vi "auto vison.vi"(3 "error in (no error)":errorcluster, 4 "Image Src":T1) -> (0 "error out":errorcluster, 1 "TOO FAR":bool, 2 "There":bool)   [LabVIEW 2014]
uses:
  <vilib>/vision/Image Controls.llb/IMAQ Image.ctl
  <vilib>/vision/NI_Vision_Development_Module.lvlib
panel:
  out "y1":dbl
  out "Image Out 2":T1(plugin-control)
  out "error out 2":errorcluster
  out "Image":T1(plugin-control)
  in  "Blue or Luma or Val or Inten Range (Find Ls)":cluster{"Lower value":i32, "Upper value":i32}={"Lower value"=84, "Upper value"=255}
  in  "Green or Sat Range (Find Ls)":cluster{"Lower value":i32, "Upper value":i32}={"Lower value"=193, "Upper value"=255}
  in  "Red or Hue Range (Find Ls)":cluster{"Lower value":i32, "Upper value":i32}={"Lower value"=79, "Upper value"=255}
  out "Image Out":T1
  out "Number of Edges (L right)":i32
  out "Edges Coordinates (L right)":cluster{"X":sgl, "Y":sgl}[](array[cluster]) {"Y" format="%.2f"; "X" format="%.2f"}
  out "Number of Edges (L left)":i32
  out "Edges Coordinates (L left)":cluster{"X":sgl, "Y":sgl}[](array[cluster]) {"Y" format="%.2f"; "X" format="%.2f"}
  out "Number of Edges (Ltop)":i32
  out "Edges Coordinates (Ltop)":cluster{"X":sgl, "Y":sgl}[](array[cluster]) {"Y" format="%.2f"; "X" format="%.2f"}
types:
  T1 = typedef "IMAQ Image.ctl" = refnum<image>
  T2 = enum16{"Get First Edge", "Get First + Last Edge", "Get All Edges"}
  T3 = cluster{"Level Type":enum32{"Absolute Value", "Relative value"}, "Threshold Level":i32, "Hysteresis":i32}
  T4 = enum32{"AutoM", "Close", "Dilate", "Erode", "Gradient", "Gradient out", "Gradient in", "Hit miss", "Open", "PClose", "POpen", "Thick", "Thin"}
  T5 = cluster{"Brightness":sgl, "Contrast":sgl, "Gamma":sgl}
  T6 = cluster{"Global Rectangle":i32[], "Contours":cluster{"ID":enum32{"External", "Internal"}, "Type":u32, "Coordinates":i32[]}[]}
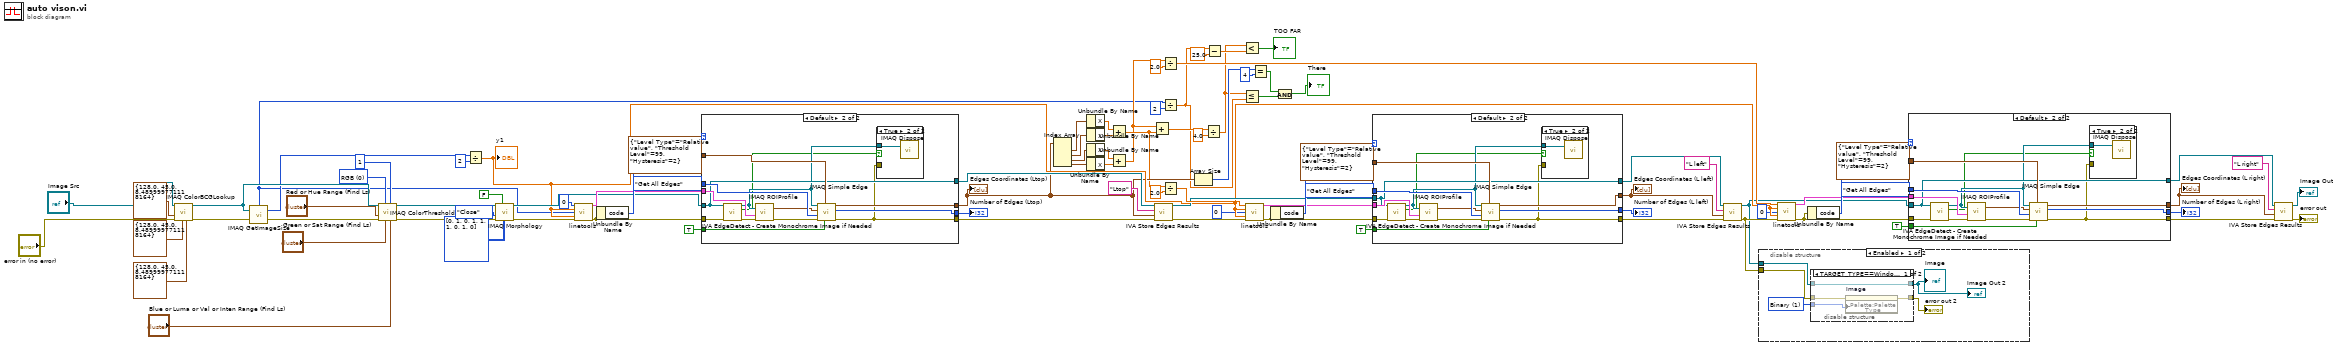
[diagram p0: block diagram]
diagram:
  w89 = u16 0 items=["RGB", "HSL", "HSV", "HSI"] ("Color Mode")
  n1 = call "IMAQ ColorBCGLookup"("Blue BCG Values"=T5 {"Brightness"=128.0, "Contrast"=45.0, "Gamma"=8.49}, "Green BCG Values"=T5 {"Brightness"=128.0, "Contrast"=45.0, "Gamma"=8.49}, "error in (no error)"="error in (no error)", "Red BCG Values"=T5 {"Brightness"=128.0, "Contrast"=45.0, "Gamma"=8.49}, "Image Src"="Image Src") -> ("error out"=w36:errorcluster, "Image Dst Out"=w56:T1)  [unwired: 2 in, 3 out]
  n2 = call "IMAQ GetImageSize"("Image"=w56, "error in (no error)"=w36) -> ("Y Resolution"=w49:i32, "X Resolution"=w14:i32, "error out"=w55:errorcluster)  [unwired: 2 in]
  n3 = call "IMAQ ColorThreshold"("Blue or Luma or Val or Inten Range"="Blue or Luma or Val or Inten Range (Find Ls)", "Replace Value"=1, "Green or Sat Range"="Green or Sat Range (Find Ls)", "Color Mode"=w89, "error in (no error)"=w55, "Red or Hue Range"="Red or Hue Range (Find Ls)", "Image Src"=w56) -> ("error out"=w34:errorcluster, "Image Dst Out"=w35:T1)  [unwired: 1 in, 2 out]
  n4 = Divide(x=w49, y=2) -> (x/y=w26:dbl)
  "y1" <- w26
  n5 = call "IMAQ Morphology"("Structuring Element"=i32[][] [[0, 1, 0], [1, 1, 1], [0, 1, 0]], "Square/Hexa (Square)"=FALSE, "error in (no error)"=w34, "Operation"=T4."Close", "Image Src"=w35) -> ("error out"=w47:errorcluster, "Image Dst Out"=w28:T1)  [unwired: 2 in, 3 out]
  n6 = call "linetools.vi"("X1"=0, "Y1"=w26, "X2"=w14, "Y2"=w26, "error in (no error)"=w47) -> ("output cluster"=w48:T6, "error out"=w29:errorcluster)  [unwired: 9 in]
  n7 = Unbundle By Name(w29) -> ("code"=w77:i32)
  n8 = case shown="Default" w77 {
    tunnel: T3 {"Level Type"=enum."Relative value", "Threshold Level"=99, "Hysteresis"=2} ("Threshold Parameters") -> [_ w108]
    tunnel: T2."Get All Edges" ("Process") -> [_ w107]
    tunnel: [_ w106] -> w80
    tunnel: w29 -> [_ w99]
    tunnel: w28 -> [w94 w100]
    tunnel: [_ w103] -> w20
    tunnel: [_ w95] -> w78
    tunnel: w48 -> [_ w102]
    tunnel: TRUE ("Sub-Pixel Accuracy") -> [_ w101]
    tunnel: [w94 w100] -> w75
    frame -1074396199, -1074396198 {
      # "Discard Coordinate System Error"
    }
    frame Default {
      n9 = call <vilib>:"IVA EdgeDetect - Create Monochrome Image if Needed.vi"("error in (no error)"=w99, "Image In"=w100) -> ("error out"=w98:errorcluster, "Mono Image Created"=w96:bool, "Mono Image Out"=w97:T1)  [unwired: 7 out]
      n10 = call "IMAQ ROIProfile"("error in (no error)"=w98, "ROI Descriptor"=w102, "Image"=w97) -> ("error out"=w104:errorcluster, "Pixel Coordinates"=w105:cluster{"X":u32, "Y":u32}[])  [unwired: 4 out]
      n11 = call "IMAQ Simple Edge"("Sub-Pixel Accuracy"=w101, "Threshold Parameters"=w108, "error in (no error)"=w104, "Process"=w107, "Pixel Coordinates"=w105, "Image Src"=w97) -> ("error out"=w95:errorcluster, "Number of Edges"=w106:i32, "Edges Coordinates"=w103:cluster{"X":sgl, "Y":sgl}[])  [unwired: 3 out]
      n12 = case shown="True" w96 {
        tunnel: w97 -> [_ w109]
        tunnel: w95 -> [_ _]
        frame False {
        }
        frame True {
          n13 = call "IMAQ Dispose"("Image"=w109) -> ()  [unwired: 2 in, 4 out]
        }
      }
    }
  }
  "Edges Coordinates (Ltop)" <- w20
  "Number of Edges (Ltop)" <- w80
  n14 = Index Array(array=w20) -> (element #1=w53:cluster{"X":sgl, "Y":sgl}, element #2=w52:cluster{"X":sgl, "Y":sgl}, element #3=w54:cluster{"X":sgl, "Y":sgl}, element #4=w51:cluster{"X":sgl, "Y":sgl})  [unwired: 4 in]
  n15 = Unbundle By Name(w53) -> ("X"=w19:sgl)
  n16 = Unbundle By Name(w52) -> ("X"=w46:sgl)
  n17 = Unbundle By Name(w54) -> ("X"=w45:sgl)
  n18 = Unbundle By Name(w51) -> ("X"=w44:sgl)
  n19 = Add(x=w19, y=w46) -> (x+y=w18:sgl)
  n20 = Add(x=w45, y=w44) -> (x+y=w17:sgl)
  n21 = Add(x=w17, y=w18) -> (x+y=w16:sgl)
  n22 = call <vilib>:"IVA Store Edges Results.vi"("error in (no error)"=w78, "Edge Coordinates"=w20, "Step Name"="Ltop", "Image in"=w75) -> ("error out"=w42:errorcluster, "Image dup"=w32:T1)  [unwired: 6 out]
  n23 = Divide(x=w17, y=sgl 2.0) -> (x/y=w27:sgl)
  n24 = Divide(x=w14, y=2) -> (x/y=w6:dbl)
  n25 = Divide(x=w18, y=sgl 2.0) -> (x/y=w41:sgl)
  n26 = Array Size(array=w20) -> (size(s)=w11:i32)
  n27 = Divide(x=w16, y=sgl 4.0) -> (x/y=w4:sgl)
  n28 = Subtract(x=w6, y=25.0) -> (x-y=w5:dbl)
  n29 = Less?(x=w4, y=w5) -> (x < y?=→"TOO FAR":bool)
  n30 = Less Or Equal?(x=w4, y=w6) -> (x <= y?=w12:bool)
  n31 = call "linetools.vi"("X1"=w41, "Y1"=w26, "X2"=0, "Y2"=w26, "error in (no error)"=w42) -> ("output cluster"=w43:T6, "error out"=w31:errorcluster)  [unwired: 9 in]
  n32 = Equal?(x=w11, y=4) -> (x = y?=w9:bool)
  n33 = Unbundle By Name(w31) -> ("code"=w68:i32)
  n34 = And(x=w9, y=w12) -> (x .and. y?=→"There":bool)
  n35 = case shown="Default" w68 {
    tunnel: T3 {"Level Type"=enum."Relative value", "Threshold Level"=99, "Hysteresis"=2} ("Threshold Parameters") -> [_ w124]
    tunnel: T2."Get All Edges" ("Process") -> [_ w123]
    tunnel: [_ w122] -> w72
    tunnel: w31 -> [_ w115]
    tunnel: w32 -> [w110 w116]
    tunnel: [_ w119] -> w70
    tunnel: [_ w111] -> w69
    tunnel: w43 -> [_ w118]
    tunnel: TRUE ("Sub-Pixel Accuracy") -> [_ w117]
    tunnel: [w110 w116] -> w66
    frame -1074396199, -1074396198 {
      # "Discard Coordinate System Error"
    }
    frame Default {
      n36 = call <vilib>:"IVA EdgeDetect - Create Monochrome Image if Needed.vi"("error in (no error)"=w115, "Image In"=w116) -> ("error out"=w114:errorcluster, "Mono Image Created"=w112:bool, "Mono Image Out"=w113:T1)  [unwired: 7 out]
      n37 = call "IMAQ ROIProfile"("error in (no error)"=w114, "ROI Descriptor"=w118, "Image"=w113) -> ("error out"=w120:errorcluster, "Pixel Coordinates"=w121:cluster{"X":u32, "Y":u32}[])  [unwired: 4 out]
      n38 = call "IMAQ Simple Edge"("Sub-Pixel Accuracy"=w117, "Threshold Parameters"=w124, "error in (no error)"=w120, "Process"=w123, "Pixel Coordinates"=w121, "Image Src"=w113) -> ("error out"=w111:errorcluster, "Number of Edges"=w122:i32, "Edges Coordinates"=w119:cluster{"X":sgl, "Y":sgl}[])  [unwired: 3 out]
      n39 = case shown="True" w112 {
        tunnel: w113 -> [_ w125]
        tunnel: w111 -> [_ _]
        frame False {
        }
        frame True {
          n40 = call "IMAQ Dispose"("Image"=w125) -> ()  [unwired: 2 in, 4 out]
        }
      }
    }
  }
  "Edges Coordinates (L left)" <- w70
  "Number of Edges (L left)" <- w72
  n41 = call <vilib>:"IVA Store Edges Results.vi"("error in (no error)"=w69, "Edge Coordinates"=w70, "Step Name"="L left", "Image in"=w66) -> ("error out"=w33:errorcluster, "Image dup"=w24:T1)  [unwired: 6 out]
  n42 = disable-structure shown="Enabled" {
    disable-tunnel: w33 -> [w127 _]
    disable-tunnel: w24 -> [w126 _]
    frame Enabled {
      w129 = u32 1 items=["Grayscale", "Binary", "Gradient", "Rainbow", "Temperature", "User Defined"] ("Palette")
      n43 = disable-structure "Conditional Disable Structure" shown="TARGET_TYPE==Windows" {
        disable-tunnel: w127 -> [w134 w135]
        disable-tunnel: [w133 w135] -> w130
        disable-tunnel: w126 -> [w132 w136]
        disable-tunnel: [w132 w136] -> w128
        disable-tunnel: w129 -> [w131 _]
        frame condition #0 {
          n44 = property on="Image" class="ImageControl"(error in=w134, "Palette:Palette Type"=w131) -> (error out=w133:errorcluster)  [unwired: 1 in, 1 out]
        }
        frame condition #1 (active) {
        }
      }
      "Image" <- w128
      "error out 2" <- w130
      "Image Out 2" <- w128
    }
    frame Disabled {
    }
  }
  n45 = call "linetools.vi"("X1"=w27, "Y1"=w26, "X2"=0, "Y2"=w26, "error in (no error)"=w33) -> ("output cluster"=w38:T6, "error out"=w23:errorcluster)  [unwired: 9 in]
  n46 = Unbundle By Name(w23) -> ("code"=w59:i32)
  n47 = case shown="Default" w59 {
    tunnel: T3 {"Level Type"=enum."Relative value", "Threshold Level"=99, "Hysteresis"=2} ("Threshold Parameters") -> [_ w151]
    tunnel: T2."Get All Edges" ("Process") -> [_ w150]
    tunnel: [_ w149] -> w63
    tunnel: w23 -> [_ w142]
    tunnel: w24 -> [w137 w143]
    tunnel: [_ w146] -> w21
    tunnel: [_ w138] -> w61
    tunnel: w38 -> [_ w145]
    tunnel: TRUE ("Sub-Pixel Accuracy") -> [_ w144]
    tunnel: [w137 w143] -> w57
    frame -1074396199, -1074396198 {
      # "Discard Coordinate System Error"
    }
    frame Default {
      n48 = call <vilib>:"IVA EdgeDetect - Create Monochrome Image if Needed.vi"("error in (no error)"=w142, "Image In"=w143) -> ("error out"=w141:errorcluster, "Mono Image Created"=w139:bool, "Mono Image Out"=w140:T1)  [unwired: 7 out]
      n49 = call "IMAQ ROIProfile"("error in (no error)"=w141, "ROI Descriptor"=w145, "Image"=w140) -> ("error out"=w147:errorcluster, "Pixel Coordinates"=w148:cluster{"X":u32, "Y":u32}[])  [unwired: 4 out]
      n50 = call "IMAQ Simple Edge"("Sub-Pixel Accuracy"=w144, "Threshold Parameters"=w151, "error in (no error)"=w147, "Process"=w150, "Pixel Coordinates"=w148, "Image Src"=w140) -> ("error out"=w138:errorcluster, "Number of Edges"=w149:i32, "Edges Coordinates"=w146:cluster{"X":sgl, "Y":sgl}[])  [unwired: 3 out]
      n51 = case shown="True" w139 {
        tunnel: w140 -> [_ w152]
        tunnel: w138 -> [_ _]
        frame False {
        }
        frame True {
          n52 = call "IMAQ Dispose"("Image"=w152) -> ()  [unwired: 2 in, 4 out]
        }
      }
    }
  }
  "Edges Coordinates (L right)" <- w21
  "Number of Edges (L right)" <- w63
  n53 = call <vilib>:"IVA Store Edges Results.vi"("error in (no error)"=w61, "Edge Coordinates"=w21, "Step Name"="L right", "Image in"=w57) -> ("error out"=→"error out":errorcluster, "Image dup"=→"Image Out":T1)  [unwired: 6 out]
